vi "Make Unsorted Group.vi"(11 "Channels":T1[](array[typedef])=[{"Name"="1", "Modbus Type"=enum."Coil", "Veristand Type"=enum."Input", "Mapping"={"DataType"=enum."Double", "Unit ID"=0, "Starting Address"=0, "Sub-Index (Bool)"=0, "VS Reference"=0}}, {"Name"="2", "Modbus Type"=enum."Coil", "Veristand Type"=enum."Input", "Mapping"={"DataType"=enum."Double", "Unit ID"=1, "Starting Address"=0, "Sub-Index (Bool)"=0, "VS Reference"=0}}, {"Name"="3", "Modbus Type"=enum."Coil", "Veristand Type"=enum."Input", "Mapping"={"DataType"=enum."Double", "Unit ID"=0, "Starting Address"=2, "Sub-Index (Bool)"=0, "VS Reference"=0}}, {"Name"="4", "Modbus Type"=enum."Coil", "Veristand Type"=enum."Input", "Mapping"={"DataType"=enum."Double", "Unit ID"=1, "Starting Address"=4, "Sub-Index (Bool)"=0, "VS Reference"=0}}] {"Mapping"."VS Reference" format="%.0x"}) -> (3 "Array":T7[](array[typedef]) {"Channel Data"."Mapping"."VS Reference" format="%.0x"})   [LabVIEW 2021, in "Modbus Master System Explorer.lvlib"]
uses:
  Modbus Master System Explorer.lvlib
  Engine/SubVIs/Bulk Data Access.ctl
  Modbus Type.ctl
  Shared/Controls/Data Model/Channel.ctl
  <vilib>/NI VeriStand/Custom Device API/Custom Device Channel Type.ctl
  Shared/Controls/Data Model/Mapping.ctl
  Shared/Controls/Data Model/DataType.ctl
  <vilib>/NI VeriStand/Custom Device API/Custom Device Item Ref.ctl
  <vilib>/NI VeriStand/Custom Device API/Custom Device API.lvlib
  Shared/Modbus Master Shared.lvlib
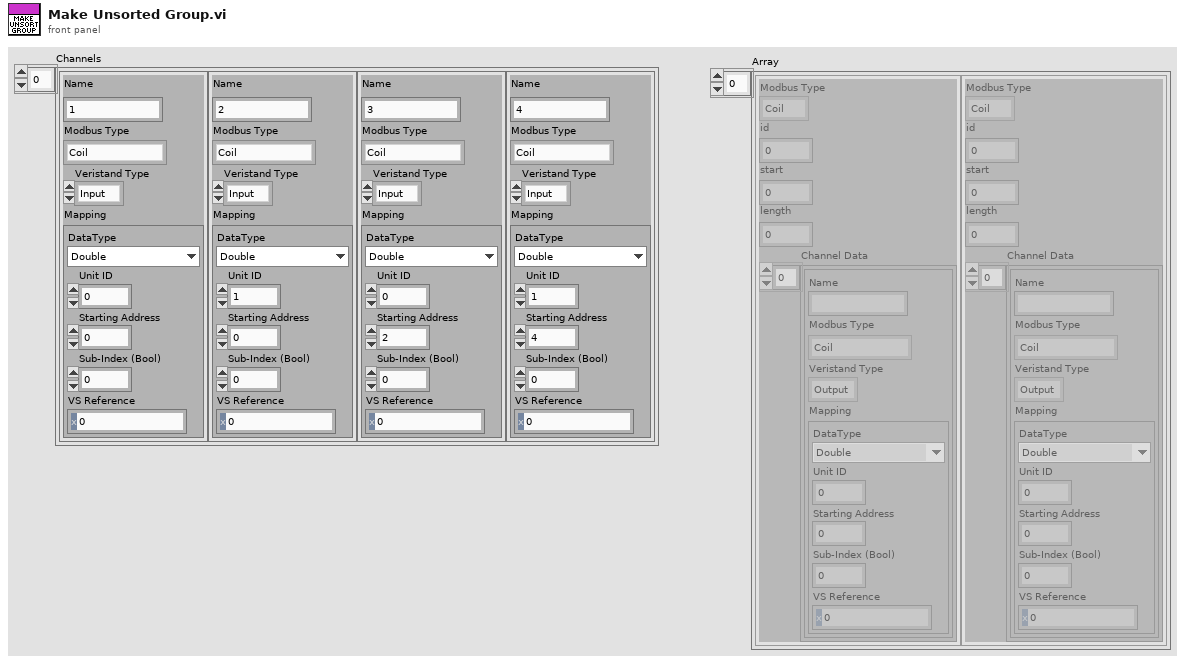
[diagram p1: front panel]
types:
  T1 = typedef "Modbus Master Shared.lvlib/Channel.ctl" = cluster{"Name":string, "Modbus Type":T2, "Veristand Type":T3, "Mapping":T4}
  T2 = typedef "Modbus Master Shared.lvlib/Modbus Type.ctl" = enum16{"Coil", "Discrete Input", "Holding Register", "Input Register"}
  T3 = typedef "Custom Device API.lvlib/Custom Device Channel Type.ctl" = enum16{"Input", "Output"}
  T4 = typedef "Modbus Master Shared.lvlib/Mapping.ctl" = cluster{"DataType":T5, "Unit ID":u8, "Starting Address":u16, "Sub-Index (Bool)":u16, "VS Reference":T6}
  T5 = typedef "Modbus Master Shared.lvlib/DataType.ctl" = enum16{"Double", "Single", "I64", "I32", "I16", "I8", "U64", "U32", "U16", "U8", "Boolean"}
  T6 = typedef "Custom Device API.lvlib/Custom Device Item Ref.ctl" = u64
  T7 = typedef "Modbus Master Shared.lvlib/Bulk Data Access.ctl" = cluster{"Modbus Type":T2, "id":u8, "start":u16, "length":u16, "Channel Data":T1[]}
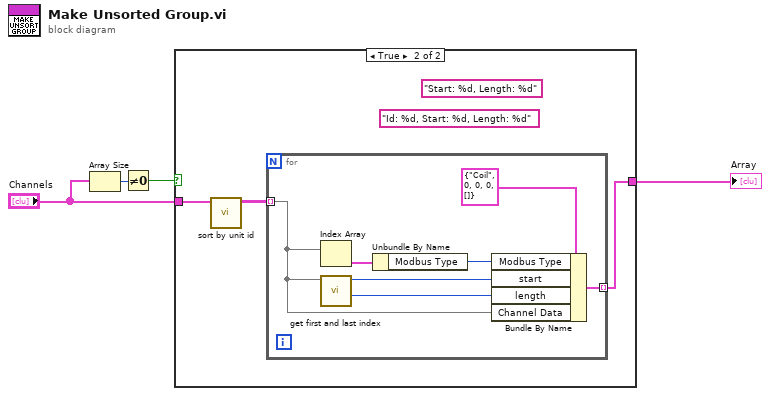
[diagram p0: block diagram]
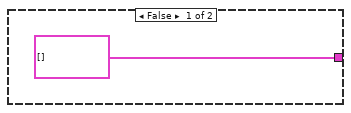
[diagram p2: hidden frame]
diagram:
  n1 = Array Size(array="Channels") -> (size(s)=w3:i32)
  n2 = Not Equal To 0?(x=w3) -> (x != 0?=w4:bool)
  n3 = case shown="True" w4 {
    tunnel: [T7[] [] w8] -> w2
    tunnel: "Channels" -> [_ w7]
    frame False {
    }
    frame True {
      (unwired) "Id: %d, Start: %d, Length: %d" ("format string")
      (unwired) "Start: %d, Length: %d" ("format string")
      n4 = call "sort by unit id.vi"("Channels"=w7) -> ("Sorted Channels"=w6:T1[][])  [unwired: 10 in]
      n5 = for {
        tunnel: [w15] -> w8 mode=indexing
        tunnel: w6 -> [w9] mode=indexing
        n6 = Index Array(array=w9) -> (element=w11:T1)  [unwired: 1 in]
        n7 = call "get first and last index.vi"("Channels In"=w9) -> ("length"=w14:u16, "Starting Register"=w13:u16)  [unwired: 8 in, 1 out]
        n8 = Unbundle By Name(w11) -> ("Modbus Type"=w10:T2)
        n9 = Bundle By Name(cluster=T7 {"Modbus Type"=enum."Coil", "id"=0, "start"=0, "length"=0, "Channel Data"=[]} ("output data access"), "Modbus Type"=w10, "start"=w13, "length"=w14, "Channel Data"=w9) -> (w15:T7)
      }
    }
  }
  "Array" <- w2
